vi "GenerateSpiralOrCircle.vi"(2 "Number of elements":dbl, 3 "Pattern running?":bool, 4 "End radius (V)":dbl, 5 "Start radius (V)":dbl) -> (0 "2D array to piezo mirror":dbl[][](array[numeric]), 1 "Output pattern (cluster)":cluster{dbl[], dbl[]})   [LabVIEW 2011]
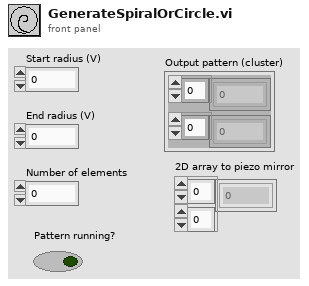
[diagram p1: front panel]
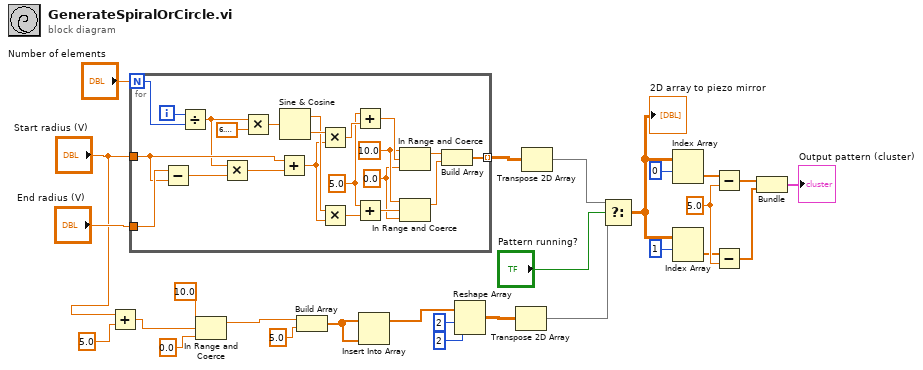
[diagram p0: block diagram]
diagram:
  w26 = 5.0 ("x")
  n1 = Add(x="Start radius (V)", y=5.0 ("x")) -> (x+y=w7:dbl)
  n2 = for {
    N: "Number of elements" -> [w48]
    tunnel: "Start radius (V)" -> [w31]
    tunnel: [w41] -> w22 mode=indexing
    tunnel: "End radius (V)" -> [w33]
    i -> [w49]
    w35 = 0.0 ("lower limit")
    w36 = 10.0 ("upper limit")
    w40 = 5.0 ("x")
    n3 = Subtract(x=w33, y=w31) -> (x-y=w32:dbl)
    n4 = Divide(x=w49, y=w48) -> (x/y=w30:dbl)
    n5 = Multiply(x=w30, y=w32) -> (x*y=w28:dbl)
    n6 = Multiply(x=w30, y=6.283185307179586) -> (x*y=w45:dbl)
    n7 = Add(x=w31, y=w28) -> (x+y=w29:dbl)
    n8 = Sine & Cosine(0:w45) -> (1:w46:dbl, 2:w47:dbl)
    n9 = Multiply(x=w47, y=w29) -> (x*y=w42:dbl)
    n10 = Multiply(x=w46, y=w29) -> (x*y=w43:dbl)
    n11 = Add(x=w40, y=w42) -> (x+y=w39:dbl)
    n12 = Add(x=w40, y=w43) -> (x+y=w37:dbl)
    n13 = In Range and Coerce(upper limit=w36, x=w39, lower limit=w35) -> (coerced(x)=w38:dbl)  [unwired: 1 out]
    n14 = In Range and Coerce(upper limit=w36, x=w37, lower limit=w35) -> (coerced(x)=w34:dbl)  [unwired: 1 out]
    n15 = Build Array(w38, w34) -> (w41:dbl[])
  }
  n16 = In Range and Coerce(upper limit=10.0, x=w7, lower limit=0.0) -> (coerced(x)=w6:dbl)  [unwired: 1 out]
  n17 = Build Array(w6, 5.0 ("element")) -> (w3:dbl[])
  n18 = Insert Into Array(array=w3, new element=w3) -> (w2:dbl[])  [unwired: 1 in]
  n19 = Reshape Array(w2, 2 ("dimension size"), 2 ("dimension size")) -> (w14:dbl[][])
  n20 = Transpose 2D Array(2D array=w14) -> (transposed array=w1:dbl[][])
  n21 = Transpose 2D Array(2D array=w22) -> (transposed array=w15:dbl[][])
  n22 = Select(t=w15, s="Pattern running?", f=w1) -> (s? t:f=w12:dbl[][])
  "2D array to piezo mirror" <- w12
  n23 = Index Array(array=w12, index (row)=0) -> (element=w20:dbl[])  [unwired: 1 in]
  n24 = Index Array(array=w12, index (row)=1) -> (element=w25:dbl[])  [unwired: 1 in]
  n25 = Subtract(x=w20, y=w26) -> (x-y=w24:dbl[])
  n26 = Subtract(x=w25, y=w26) -> (x-y=w27:dbl[])
  n27 = Bundle(w24, w27) -> (→"Output pattern (cluster)":cluster{dbl[], dbl[]})  [unwired: 1 in]
